vi "Comments.Create Lockin REF Description.vi"(7 "error in (no error)":errorcluster, 10 "Control Experiment":refnum<class "Control Experiment.lvclass">) -> (0 "error out":errorcluster, 2 "REF Section":string, 3 "Control Experiment out":refnum<class "Control Experiment.lvclass">)   [LabVIEW 2016, in "Control Experiment.lvclass"]
uses:
  Control Experiment.lvclass
  <userlib>/LevyLab/Lockin-Multichannel/Instrument.Lockin/Instrument.Lockin.lvclass
  <userlib>/LevyLab/PLYM/YAML.lvclass
  C:/Program Files (x86)/National Instruments/LabVIEW 2016/user.lib/LevyLab/Levylab Instruments/SMOs/Instrument/Instrument.lvclass
  C:/Program Files (x86)/National Instruments/LabVIEW 2016/vi.lib/JKI/JKI SMO/SMO/SMO.lvclass
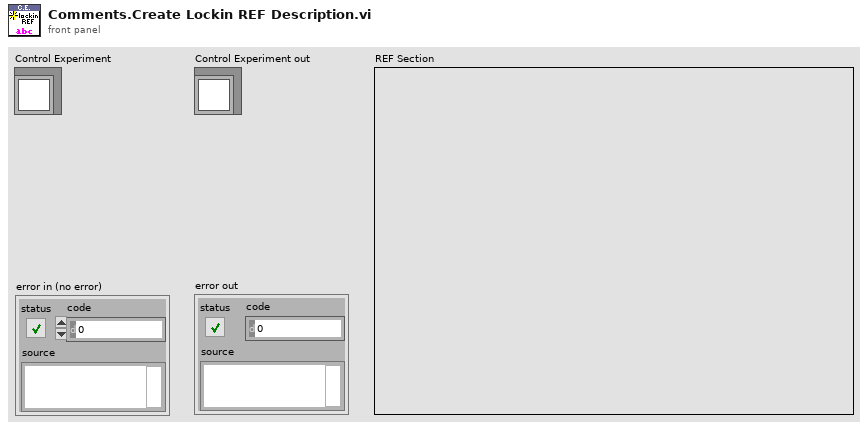
[diagram p1: front panel]
types:
  T1 = typedef "Lockin.DAQ.lvclass/REF-cluster.ctl" = T2[]
  T2 = typedef "Instrument.Lockin.UI.lvclass/REF Channel--Cluster.ctl" = cluster{"Enable?":bool, "Channel":i32, "Frequency":dbl, "Phase":dbl, "TC":dbl, "Order":i32}
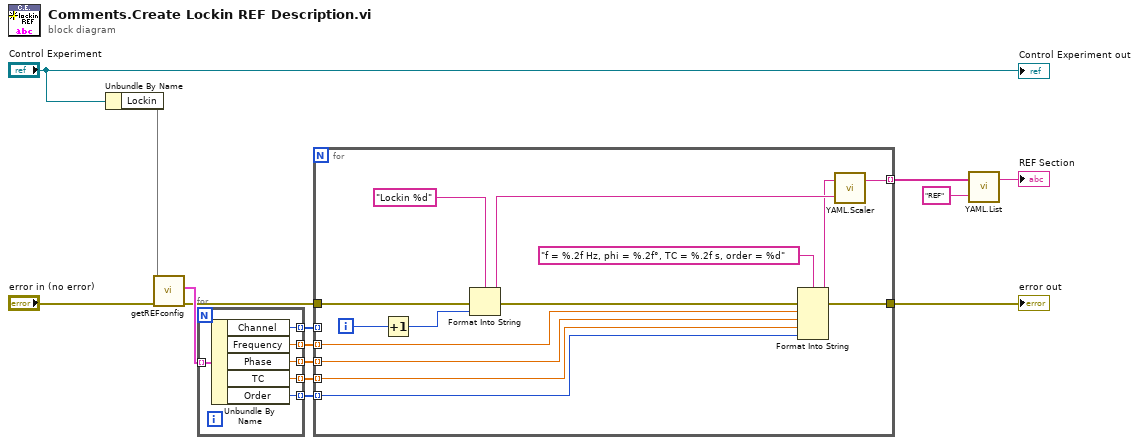
[diagram p0: block diagram]
diagram:
  n1 = Unbundle By Name("Control Experiment") -> ("Lockin"=w5)
  n2 = call <userlib>:"getREFconfig.vi"("error in (no error)"="error in (no error)", "Instrument.Lockin in"=w5) -> ("error out"=w4:errorcluster, "REFconfig"=w6:T1)  [unwired: 7 in, 1 out]
  n3 = for {
    tunnel: [w20] -> w14 mode=indexing
    tunnel: [w19] -> w13 mode=indexing
    tunnel: w6 -> [w18] mode=indexing
    tunnel: [w17] -> w3 mode=indexing
    tunnel: [w16] -> w2 mode=indexing
    tunnel: [w15] -> w1 mode=indexing
    n4 = Unbundle By Name(w18) -> ("Channel"=w20:i32, "Frequency"=w19:dbl, "Phase"=w17:dbl, "TC"=w16:dbl, "Order"=w15:i32)
  }
  n5 = for {
    tunnel: w14 -> [_] mode=indexing
    tunnel: w13 -> [w25] mode=indexing
    tunnel: w4 -> [w34]
    tunnel: [w33] -> w12
    tunnel: [w27] -> w7 mode=indexing
    tunnel: w3 -> [w24] mode=indexing
    tunnel: w2 -> [w23] mode=indexing
    tunnel: w1 -> [w22] mode=indexing
    i -> [w32]
    n6 = Increment(x=w32) -> (x+1=w26:i32)
    n7 = Format Into String(format string="Lockin %d", error in=w34, w26) -> (resulting string=w28:string, error out=w29:errorcluster)  [unwired: 1 in]
    n8 = Format Into String(format string="f = %.2f Hz, phi = %.2f°, TC = %.2f s, order = %d", error in=w29, w25, w24, w23, w22) -> (resulting string=w21:string, error out=w33:errorcluster)  [unwired: 1 in]
    n9 = call <userlib>:"YAML.Scaler.vi"("Key"=w28, "Scaler"=w21) -> ("Output"=w27:string)  [unwired: 1 in]
  }
  "error out" <- w12
  n10 = call <userlib>:"YAML.List.vi"("Key"="REF" ("string"), "lines"=w7) -> ("Output"=→"REF Section":string)  [unwired: 1 in]
  "Control Experiment out" <- "Control Experiment"
